vi "Pose3d_NearestTo.vi"(9 "other POSE3d":T1[](array[typedef]) {"Translation3d"."Z" format="%14.3f"; "Translation3d"."Y" format="%14.3f"; "Translation3d"."X" format="%14.3f"}, 11 "in POSE3d":T1={"Translation3d"={"X"=0.0, "Y"=0.0, "Z"=0.0}, "Rotation3d"={"Q_quaternion"={"R"=1.0, "V"=[0.0, 0.0, 0.0]}}} {"Translation3d"."Z" format="%14.3f"; "Translation3d"."Y" format="%14.3f"; "Translation3d"."X" format="%14.3f"}) -> (1 "Found":bool, 3 "Nearest Pose3d":T1={"Translation3d"={"X"=0.0, "Y"=0.0, "Z"=0.0}, "Rotation3d"={"Q_quaternion"={"R"=1.0, "V"=[0.0, 0.0, 0.0]}}} {"Translation3d"."Z" format="%14.3f"; "Translation3d"."Y" format="%14.3f"; "Translation3d"."X" format="%14.3f"})   [LabVIEW 2019, in "Trajectory_Library.lvlib"]
doc: "Returns the Transform2d that maps the one pose to another.\n\nParameter:\n - IN POSE - Current POSE data structure\n - OTHER POSE - The initial pose of the transformation.\n\nReturns:\n - OUT TRANSFORMATION - The transform that maps the other pose to the current pose."
uses:
  Trajectory_Library.lvlib
  TypeDef/TRANSLATION3D.ctl
  TypeDef/QUATERNION.ctl
  TypeDef/ROTATION3D.ctl
  TypeDef/POSE3D.ctl
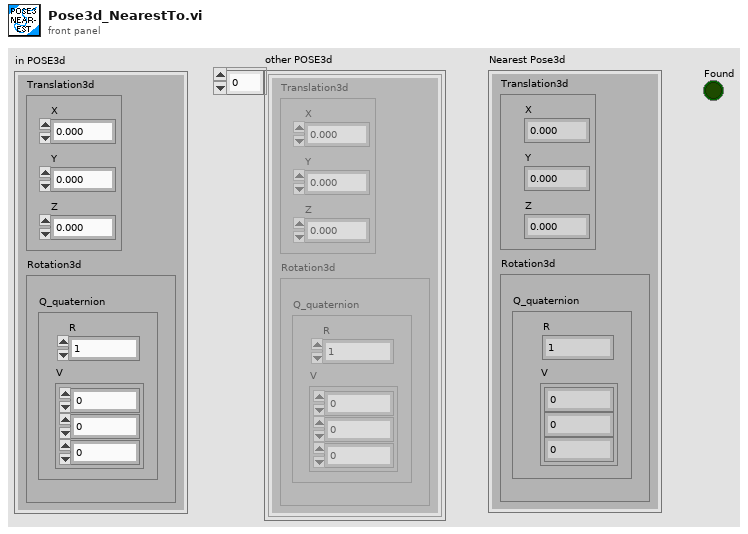
[diagram p1: front panel]
types:
  T1 = typedef "Trajectory_Library.lvlib/POSE3D.ctl" = cluster{"Translation3d":T2, "Rotation3d":T3}
  T2 = typedef "Trajectory_Library.lvlib/TRANSLATION3D.ctl" = cluster{"X":dbl, "Y":dbl, "Z":dbl}
  T3 = typedef "Trajectory_Library.lvlib/ROTATION3D.ctl" = cluster{"Q_quaternion":T4}
  T4 = typedef "Trajectory_Library.lvlib/QUATERNION.ctl" = cluster{"R":dbl, "V":dbl[]}
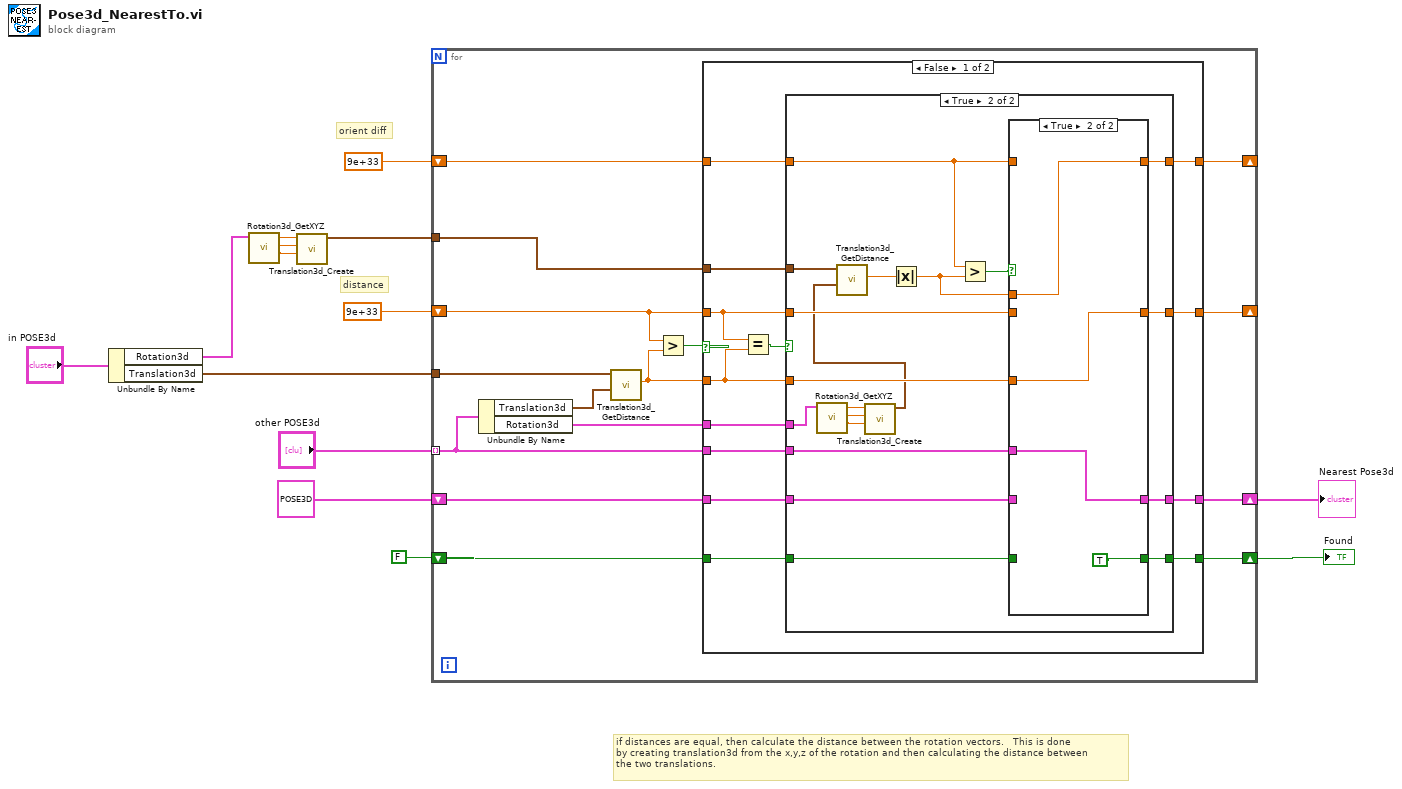
[diagram p0: block diagram]
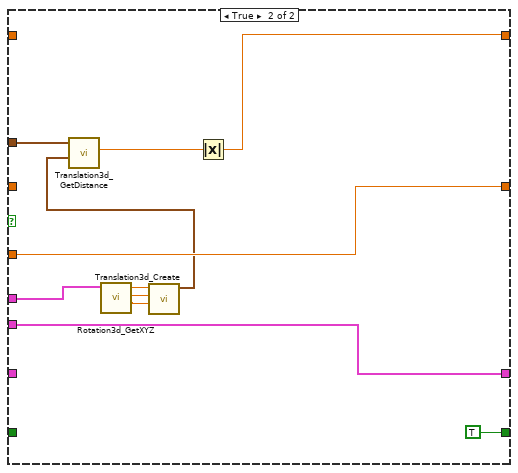
[diagram p4: hidden frame]
diagram:
  # "if distances are equal, then calculate the distance between the rotation vectors.   This is done\nby creating translation3d from the x,y,z of the rotation and then calculating the distance between\nthe two translations."
  # "orient diff"
  # "distance"
  n1 = Unbundle By Name("in POSE3d") -> ("Rotation3d"=w5:T3, "Translation3d"=w6:T2)
  n2 = call "Rotation3d_GetXYZ.vi"("in Rotation3d"=w5) -> ("Z"=w2:dbl, "Y"=w3:dbl, "X"=w4:dbl)  [unwired: 8 in]
  n3 = call "Translation3d_Create.vi"("Z"=w2, "Y"=w3, "X"=w4) -> ("TRANSLATION3D"=w1:T2)  [unwired: 8 in]
  n4 = for {
    shift-right: [w28] -> _
    shift-left: 9e+33 -> [w24]
    tunnel: "other POSE3d" -> [w21] mode=indexing
    shift-right: [w25] -> w9
    shift-left: FALSE -> [w22]
    shift-right: [w26] -> w10
    shift-left: T1 {"Translation3d"={"X"=0.0, "Y"=0.0, "Z"=0.0}, "Rotation3d"={"Q_quaternion"={"R"=1.0, "V"=[0.0, 0.0, 0.0]}}} ("other POSE") -> [w23]
    shift-right: [w18] -> _
    shift-left: 9e+33 -> [w19]
    tunnel: w6 -> [w16]
    tunnel: w1 -> [w15]
    n5 = Unbundle By Name(w21) -> ("Translation3d"=w20:T2, "Rotation3d"=w17:T3)
    n6 = call "Translation3d_GetDistance.vi"("other Translation3d"=w20, "In Translation3d"=w16) -> ("Distance"=w27:dbl)  [unwired: 9 in]
    n7 = Greater?(x=w24, y=w27) -> (0:w29:bool)
    n8 = case shown="False" w29 {
      tunnel: w21 -> [w31 w83]
      tunnel: [w40 w84] -> w28
      tunnel: w27 -> [w32 w84]
      tunnel: [w37 w83] -> w26
      tunnel: [w36 TRUE] -> w25
      tunnel: w24 -> [w41 _]
      tunnel: w23 -> [w38 _]
      tunnel: w22 -> [w39 _]
      tunnel: w19 -> [w35 _]
      tunnel: [w34 w81] -> w18
      tunnel: w17 -> [w33 w77]
      tunnel: w15 -> [w30 w76]
      frame False {
        n9 = Equal?(x=w41, y=w32) -> (x = y?=w42:bool)
        n10 = case shown="True" w42 {
          tunnel: w41 -> [w46 w56]
          tunnel: [w46 w62] -> w40
          tunnel: w39 -> [w44 w54]
          tunnel: w38 -> [w45 w55]
          tunnel: [w45 w60] -> w37
          tunnel: [w44 w58] -> w36
          tunnel: w35 -> [w43 w57]
          tunnel: [w43 w64] -> w34
          tunnel: w33 -> [_ w50]
          tunnel: w32 -> [_ w61]
          tunnel: w31 -> [_ w59]
          tunnel: w30 -> [_ w48]
          frame False {
          }
          frame True {
            n11 = call "Rotation3d_GetXYZ.vi"("in Rotation3d"=w50) -> ("Z"=w51:dbl, "Y"=w52:dbl, "X"=w53:dbl)  [unwired: 8 in]
            n12 = call "Translation3d_Create.vi"("Z"=w51, "Y"=w52, "X"=w53) -> ("TRANSLATION3D"=w49:T2)  [unwired: 8 in]
            n13 = call "Translation3d_GetDistance.vi"("other Translation3d"=w49, "In Translation3d"=w48) -> ("Distance"=w47:dbl)  [unwired: 9 in]
            n14 = Absolute Value(x=w47) -> (abs(x)=w63:dbl)
            n15 = Greater?(x=w57, y=w63) -> (0:w65:bool)
            n16 = case shown="True" w65 {
              tunnel: [w69 w73] -> w64
              tunnel: w63 -> [_ w73]
              tunnel: [w68 w72] -> w62
              tunnel: w61 -> [_ w72]
              tunnel: [w67 w71] -> w60
              tunnel: w59 -> [_ w71]
              tunnel: [w66 TRUE] -> w58
              tunnel: w57 -> [w69 _]
              tunnel: w56 -> [w68 _]
              tunnel: w55 -> [w67 _]
              tunnel: w54 -> [w66 _]
              frame False {
              }
              frame True {
              }
            }
          }
        }
      }
      frame True {
        n17 = call "Rotation3d_GetXYZ.vi"("in Rotation3d"=w77) -> ("Z"=w78:dbl, "Y"=w79:dbl, "X"=w80:dbl)  [unwired: 8 in]
        n18 = call "Translation3d_Create.vi"("Z"=w78, "Y"=w79, "X"=w80) -> ("TRANSLATION3D"=w75:T2)  [unwired: 8 in]
        n19 = call "Translation3d_GetDistance.vi"("other Translation3d"=w75, "In Translation3d"=w76) -> ("Distance"=w74:dbl)  [unwired: 9 in]
        n20 = Absolute Value(x=w74) -> (abs(x)=w81:dbl)
      }
    }
  }
  "Nearest Pose3d" <- w10
  "Found" <- w9
